vi "fit_parameters_chooser.vi"(0 "Physical constants refnum":refnum<vi>, 1 "C refnum":refnum<vi>, 2 "Fit parameters refnum":refnum<vi>, 3 "Stop notification queue":refnum<queue>) -> ()   [LabVIEW 2015]
uses:
  fit_parameters.ctl
  physical_constants.ctl
  <vilib>/gmath/statdist.llb/Continuous PDF.vi
  <vilib>/gmath/statdist.llb/Normal PDF.vi
  <vilib>/gmath/NI_Gmath.lvlib
panel:
  in  "Refresh graphs":bool
  in  "Use experimental values":bool
  in  "Update simulation parameters":bool
  in  "Physical constants":T1={"T1e (s)"=0.03, "T1n (s)"=1500.0}
  in  "C":dbl=0.000136073
  in  "Fit parameters":T2={"A"=0.572086, "S"=0.0835606, "M1"=140.286, "M2"=140.486}
  out "Steady state distribution":cluster{dbl[], dbl[]}(graph)
  out "Alpha/beta distributions":cluster{dbl[], dbl[]}[](graph)
  # "Explanation of fit parameters:\nThe parameters A, S, M1, and M2 control the distribution of alpha and beta as shown above. The steady state distribution will be computed from these.\nA: the height of the Gaussian distributions for alpha and beta\nS: the standard deviation of the Gaussian distributions for alpha and beta\nM1: the mean of the Gaussian distribution for beta\nM2: the mean of the Gaussian distribution for alpha"
  # "Internal controls"
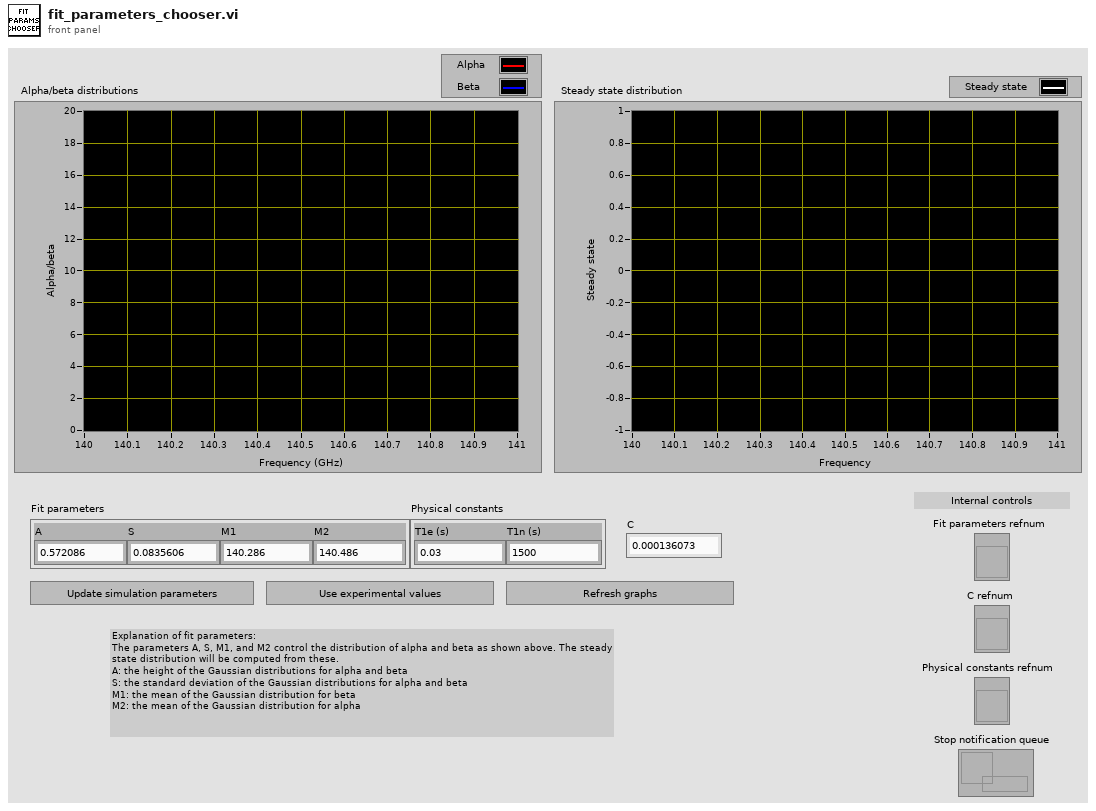
[diagram p1: front panel]
types:
  T1 = typedef "physical_constants.ctl" = cluster{"T1e (s)":dbl, "T1n (s)":dbl}
  T2 = typedef "fit_parameters.ctl" = cluster{"A":dbl, "S":dbl, "M1":dbl, "M2":dbl}
  T3 = typedef "LVRangeTypeDef.ctl" = cluster{"Minimum":dbl, "Maximum":dbl, "Increment":dbl, "Minor Increment":dbl, "Start":dbl}
  T4 = enum8{"Enabled", "Disabled", "Disabled and Grayed Out"}
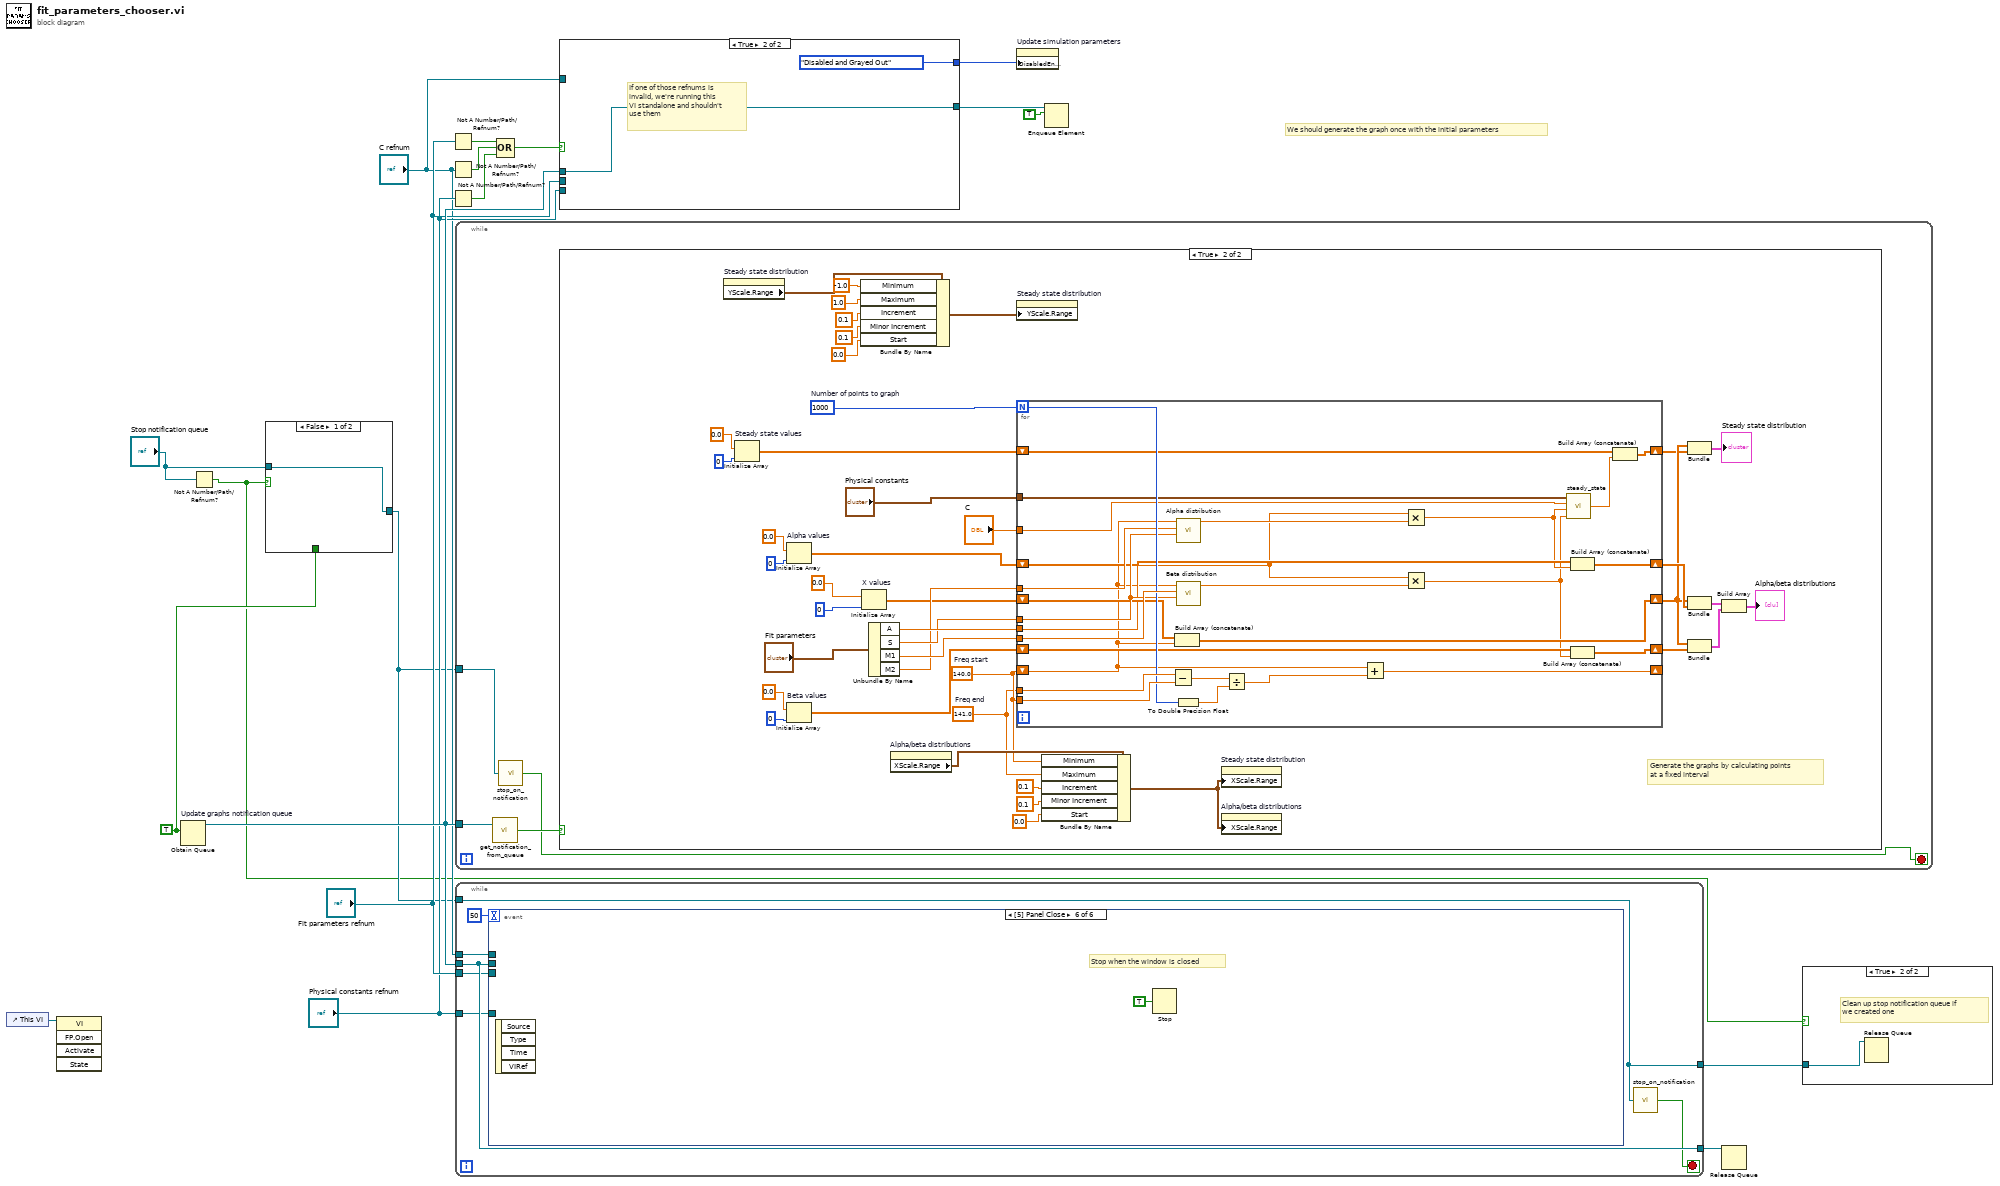
[diagram p0: block diagram]
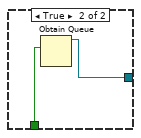
[diagram p3: hidden frame]
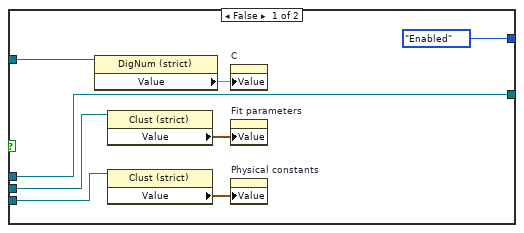
[diagram p4: hidden frame]
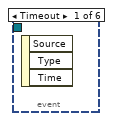
[diagram p5: hidden frame]
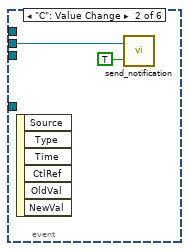
[diagram p6: hidden frame]
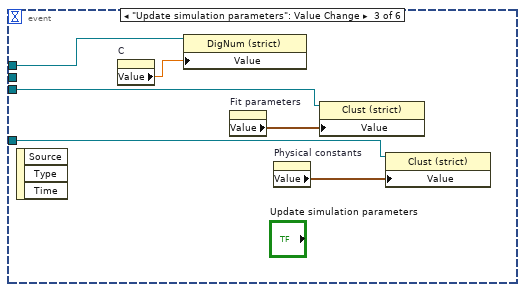
[diagram p7: hidden frame]
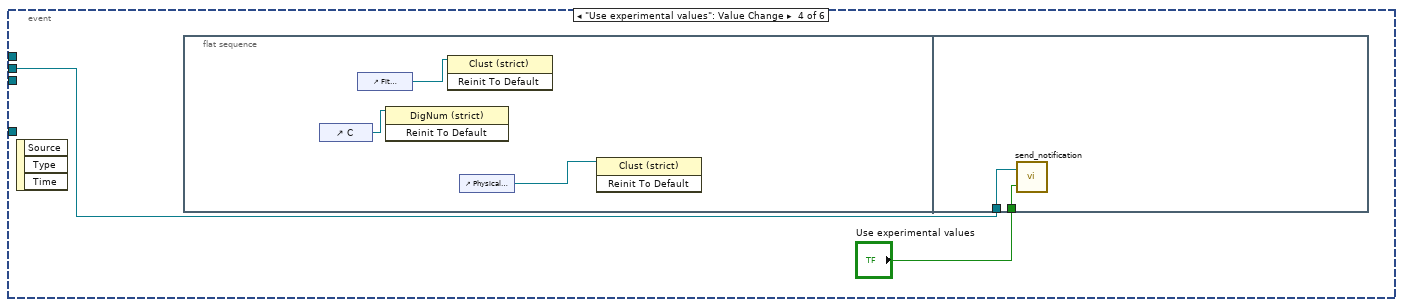
[diagram p8: hidden frame]
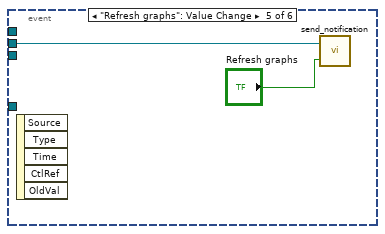
[diagram p9: hidden frame]
diagram:
  w6 = TRUE
  # "We should generate the graph once with the initial parameters"
  n1 = control-ref of="This VI"() -> (w1:refnum<vi>)
  n2 = invoke class="VI" method="FP.Open"(reference=w1) -> ()  [unwired: 4 in, 5 out]
  n3 = Obtain Queue "Update graphs notification queue"(element data type=w6) -> (queue out=w11:refnum<queue>)  [unwired: 4 in, 2 out]
  n4 = Not A Number/Path/Refnum?(number/path/refnum="Stop notification queue") -> (NaN/Path/Refnum?=w3:bool)
  n5 = case shown="False" w3 {
    tunnel: w6 -> [_ w21]
    tunnel: [w19 w20] -> w4
    tunnel: "Stop notification queue" -> [w19 _]
    frame False {
    }
    frame True {
      n6 = Obtain Queue(element data type=w21) -> (queue out=w20:refnum<queue>)  [unwired: 4 in, 2 out]
    }
  }
  n7 = Not A Number/Path/Refnum?(number/path/refnum="Fit parameters refnum") -> (NaN/Path/Refnum?=w16:bool)
  n8 = Not A Number/Path/Refnum?(number/path/refnum="C refnum") -> (NaN/Path/Refnum?=w15:bool)
  n9 = Not A Number/Path/Refnum?(number/path/refnum="Physical constants refnum") -> (NaN/Path/Refnum?=w14:bool)
  n10 = while {
    tunnel: w11 -> [w24]
    tunnel: w4 -> [w23]
    stop <- w22 stop-if-true
    n11 = call "get_notification_from_queue.vi"("Queue in"=w24) -> ("Should act"=w25:bool)  [unwired: 1 in, 2 out]
    n12 = call "stop_on_notification.vi"("Notofication queue"=w23) -> ("Should stop"=w22:bool)
    n13 = case shown="True" w25 {
      frame False {
      }
      frame True {
        w60 = 141.0  # Freq end
        w61 = 140.0  # Freq start
        w66 = 1000  # Number of points to graph
        # "Generate the graphs by calculating points\nat a fixed interval"
        n14 = property on="Steady state distribution" class="XYGraph (strict)"() -> ("YScale.Range"=w32:T3)  [unwired: 2 in, 2 out]
        n15 = Initialize Array "Steady state values"(0.0 ("element"), 0 ("dimension size")) -> (w38:dbl[])
        n16 = Initialize Array "Alpha values"(0.0 ("element"), 0 ("dimension size")) -> (w47:dbl[])
        n17 = Initialize Array "Beta values"(0.0 ("element"), 0 ("dimension size")) -> (w48:dbl[])
        n18 = Bundle By Name(cluster=w32, "Minimum"=-1.0, "Maximum"=1.0, "Increment"=0.1, "Minor Increment"=0.1, "Start"=0.0) -> (w31:T3)
        n19 = Initialize Array "X values"(0.0 ("element"), 0 ("dimension size")) -> (w53:dbl[])
        n20 = Unbundle By Name("Fit parameters") -> ("A"=w65:dbl, "S"=w63:dbl, "M1"=w64:dbl, "M2"=w56:dbl)
        n21 = property on="Alpha/beta distributions" class="XYGraph (strict)"() -> ("XScale.Range"=w62:T3)  [unwired: 2 in, 2 out]
        n22 = property on="Steady state distribution" class="XYGraph (strict)"("YScale.Range"=w31) -> ()  [unwired: 2 in, 2 out]
        n23 = for {
          N: w66 -> [w88]
          shift-right: [w86] -> _
          shift-left: w61 -> [w75]
          tunnel: w65 -> [w79]
          tunnel: w64 -> [w93]
          tunnel: w63 -> [w84]
          tunnel: w60 -> [w92]
          tunnel: w61 -> [w91]
          tunnel: w56 -> [w85]
          shift-right: [w76] -> w37
          shift-left: w53 -> [w83]
          shift-right: [w78] -> w45
          shift-left: w48 -> [w81]
          shift-right: [w77] -> w46
          shift-left: w47 -> [w82]
          shift-right: [w72] -> w36
          shift-left: w38 -> [w74]
          tunnel: "Physical constants" -> [w71]
          tunnel: "C" -> [w70]
          n24 = Subtract(x=w92, y=w91) -> (x-y=w90:dbl)
          n25 = Build Array (concatenate)(w83, w75) -> (w76:dbl[])
          n26 = call-poly "Alpha distribution"("std"=w84, "mean"=w85, "x"=w75) -> ("pdf(x)"=w80:dbl)  [unwired: 7 in, 1 out]
          n27 = call-poly "Beta distribution"("std"=w84, "mean"=w93, "x"=w75) -> ("pdf(x)"=w94:dbl)  [unwired: 7 in, 1 out]
          n28 = To Double Precision Float(number=w88) -> (double precision float=w89:dbl)
          n29 = Divide(x=w90, y=w89) -> (x/y=w87:dbl)
          n30 = Add(x=w75, y=w87) -> (x+y=w86:dbl)
          n31 = Multiply(x=w79, y=w80) -> (x*y=w69:dbl)
          n32 = Multiply(x=w79, y=w94) -> (x*y=w68:dbl)
          n33 = call "steady_state.vi"("Beta"=w68, "Alpha"=w69, "C"=w70, "Physical constants"=w71) -> ("Steady state"=w73:dbl)
          n34 = Build Array (concatenate)(w82, w69) -> (w77:dbl[])
          n35 = Build Array (concatenate)(w81, w68) -> (w78:dbl[])
          n36 = Build Array (concatenate)(w74, w73) -> (w72:dbl[])
        }
        n37 = Bundle By Name(cluster=w62, "Minimum"=w61, "Maximum"=w60, "Increment"=0.1, "Minor Increment"=0.1, "Start"=0.0) -> (w41:T3)
        n38 = property on="Steady state distribution" class="XYGraph (strict)"("XScale.Range"=w41) -> ()  [unwired: 2 in, 2 out]
        n39 = property on="Alpha/beta distributions" class="XYGraph (strict)"("XScale.Range"=w41) -> ()  [unwired: 2 in, 2 out]
        n40 = Bundle(w37, w36) -> (→"Steady state distribution":cluster{dbl[], dbl[]})  [unwired: 1 in]
        n41 = Bundle(w37, w46) -> (w44:cluster{dbl[], dbl[]})  [unwired: 1 in]
        n42 = Bundle(w37, w45) -> (w43:cluster{dbl[], dbl[]})  [unwired: 1 in]
        n43 = Build Array(w44, w43) -> (→"Alpha/beta distributions":cluster{dbl[], dbl[]}[])
      }
    }
  }
  n44 = while {
    tunnel: w11 -> [w101]
    tunnel: [w101] -> w18
    tunnel: "Fit parameters refnum" -> [w100]
    tunnel: "Physical constants refnum" -> [w99]
    tunnel: "C refnum" -> [w98]
    tunnel: w4 -> [w96]
    tunnel: [w96] -> w2
    stop <- w97 stop-if-true
    n45 = event shown="[5] Panel Close" {
      selector: _ -> [_ _ _ _ _ _]
      dyn-events: _ -> [_ _ _ _ _ _]
      timeout: 50 -> [_ _ _ _ _ _]
      tunnel: w101 -> [_ w103 _ w111 w117 _]
      tunnel: w100 -> [_ _ w109 _ _ _]
      tunnel: w99 -> [_ _ w108 _ _ _]
      tunnel: w98 -> [_ _ w107 _ _ _]
      event Timeout {
        n46 = event-data() -> ()  [unwired: 1 in, 3 out]
      }
      event "C": Value Change {
        n47 = event-data() -> ()  [unwired: 1 in, 6 out]
        n48 = call "send_notification.vi"("Notification"=TRUE, "Notification queue in"=w103) -> ()  [unwired: 1 out]
      }
      event "Update simulation parameters": Value Change {
        n49 = event-data() -> ()  [unwired: 1 in, 3 out]
        n50 = property on="C" class="DigNum (strict)"() -> ("Value"=w104:dbl)  [unwired: 2 in, 2 out]
        n51 = property class="DigNum (strict)"(reference=w107, "Value"=w104) -> ()  [unwired: 1 in, 2 out]
        n52 = property on="Fit parameters" class="Clust (strict)"() -> ("Value"=w106:T2)  [unwired: 2 in, 2 out]
        n53 = property on="Physical constants" class="Clust (strict)"() -> ("Value"=w105:T1)  [unwired: 2 in, 2 out]
        n54 = property class="Clust (strict)"(reference=w109, "Value"=w106) -> ()  [unwired: 1 in, 2 out]
        n55 = property class="Clust (strict)"(reference=w108, "Value"=w105) -> ()  [unwired: 1 in, 2 out]
      }
      event "Use experimental values": Value Change {
        n56 = event-data() -> ()  [unwired: 1 in, 3 out]
        n57 = flat-sequence {
          tunnel: w111 -> [w116]
          tunnel: "Use experimental values" -> [w115]
          frame #0 {
            n58 = control-ref of="C"() -> (w112:refnum<vi>)
            n59 = control-ref of="Fit parameters"() -> (w114:refnum<vi>)
            n60 = invoke class="DigNum (strict)" method="Reinit To Default"(reference=w112) -> ()  [unwired: 2 in, 3 out]
            n61 = invoke class="Clust (strict)" method="Reinit To Default"(reference=w114) -> ()  [unwired: 2 in, 3 out]
            n62 = control-ref of="Physical constants"() -> (w113:refnum<vi>)
            n63 = invoke class="Clust (strict)" method="Reinit To Default"(reference=w113) -> ()  [unwired: 2 in, 3 out]
          }
          frame #1 {
            n64 = call "send_notification.vi"("Notification"=w115, "Notification queue in"=w116) -> ()  [unwired: 1 out]
          }
        }
      }
      event "Refresh graphs": Value Change {
        n65 = event-data() -> ()  [unwired: 1 in, 5 out]
        n66 = call "send_notification.vi"("Notification"="Refresh graphs", "Notification queue in"=w117) -> ()  [unwired: 1 out]
      }
      event Panel Close {
        # "Stop when the window is closed"
        n67 = event-data() -> ()  [unwired: 1 in, 4 out]
        n68 = Stop(stop? (T)=TRUE) -> ()
      }
    }
    n69 = call "stop_on_notification.vi"("Notofication queue"=w96) -> ("Should stop"=w97:bool)
  }
  n70 = Compound Arithmetic op=OR(w16, w15, w14) -> (w17:bool)
  n71 = case shown="True" w17 {
    tunnel: [T4."Enabled" ("Disabled") T4."Disabled and Grayed Out" ("Disabled")] -> w13
    tunnel: "Fit parameters refnum" -> [w126 _]
    tunnel: "C refnum" -> [w124 _]
    tunnel: "Physical constants refnum" -> [w123 _]
    tunnel: w11 -> [w120 w128]
    tunnel: [w120 w128] -> w10
    frame False {
      n72 = property class="DigNum (strict)"(reference=w124) -> ("Value"=w122:dbl)  [unwired: 1 in, 2 out]
      n73 = property class="Clust (strict)"(reference=w126) -> ("Value"=w125:T2)  [unwired: 1 in, 2 out]
      n74 = property class="Clust (strict)"(reference=w123) -> ("Value"=w121:T1)  [unwired: 1 in, 2 out]
      n75 = property on="C" class="DigNum (strict)"("Value"=w122) -> ()  [unwired: 2 in, 2 out]
      n76 = property on="Fit parameters" class="Clust (strict)"("Value"=w125) -> ()  [unwired: 2 in, 2 out]
      n77 = property on="Physical constants" class="Clust (strict)"("Value"=w121) -> ()  [unwired: 2 in, 2 out]
    }
    frame True {
      # "If one of those refnums is\ninvalid, we're running this\nVI standalone and shouldn't\nuse them"
    }
  }
  n78 = property on="Update simulation parameters" class="Bool"("DisabledEnum"=w13) -> ()  [unwired: 2 in, 2 out]
  n79 = Enqueue Element(queue=w10, element=TRUE) -> ()  [unwired: 2 in, 3 out]
  n80 = Release Queue(queue=w18) -> ()  [unwired: 2 in, 3 out]
  n81 = case shown="True" w3 {
    tunnel: w2 -> [_ w130]
    frame False {
    }
    frame True {
      # "Clean up stop notification queue if\nwe created one"
      n82 = Release Queue(queue=w130) -> ()  [unwired: 2 in, 3 out]
    }
  }
